vi "Launch.vi"(8 "error in (no error)":errorcluster, 9 "Interface Thread Parameters":refnum<class "Thread Parameters.lvclass">, 10 "Work Thread Parameters":refnum<class "Thread Parameters.lvclass">, 11 "Dispatcher in":refnum<class "Dispatcher.lvclass">) -> (0 "error out":errorcluster, 3 "Dispatcher out":refnum<class "Dispatcher.lvclass">)   [LabVIEW 2017, in "DSF Core.lvlib" / "Dispatcher.lvclass"]
uses:
  Dispatcher.lvclass
  Thread Parameters/Thread Parameters.lvclass
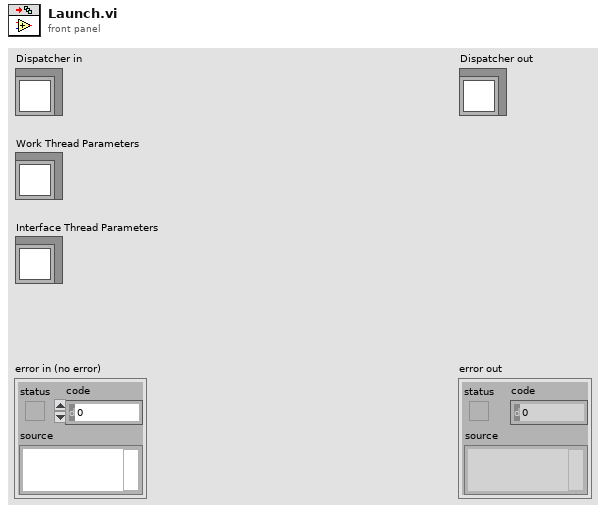
[diagram p1: front panel]
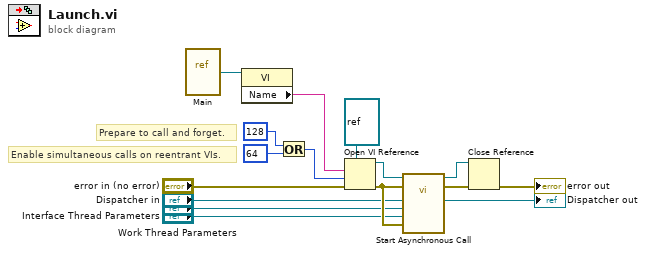
[diagram p0: block diagram]
diagram:
  # "Prepare to call and forget."
  # "Enable simultaneous calls on reentrant VIs."
  n1 = vi-ref "Main.vi"() -> (w5:refnum<vi>)
  n2 = property class="VI"(reference=w5) -> ("Name"=w4:string)  [unwired: 1 in, 2 out]
  n3 = Or(x=128 ("options"), y=64 ("options")) -> (x .or. y?=w8:i32)
  n4 = Open VI Reference(type specifier VI Refnum (for type only)=refnum<vi> refnum, vi path=w4, options=w8, error in (no error)="error in (no error)") -> (vi reference=w13:refnum<vi>, error out=w15:errorcluster)  [unwired: 2 in]
  n5 = call-by-ref "Start Asynchronous Call"(reference=w13, error in=w15, 8:"error in (no error)"=w15, "Dispatcher Interface Thread Parameters"="Interface Thread Parameters", "Dispatcher Work Thread Parameters"="Work Thread Parameters", "Dispatcher in"="Dispatcher in") -> (reference out=w11:refnum<vi>, error out=w12:errorcluster)  [unwired: 6 in, 2 out]
  n6 = Close Reference(reference=w11, error in (no error)=w12) -> (error out=→"error out":errorcluster)
  "Dispatcher out" <- "Dispatcher in"
